vi "FFT_Austin.vi"() -> ()   [LabVIEW 2021]
uses:
  <vilib>/rvi/DataTransferAndStorage/Container/XNode/niFpgaContainer.xnode
  <vilib>/rvi/interface/RandomDataEmulation/nirviRandomDataFpgaReadWriteTemplate.vi
  <vilib>/rvi/Analysis/measure/FFT/XNode/niFpgaFFT.xnode
  <vilib>/rvi/LocalResourceManager/LocalResourceManager.xnode
  <vilib>/rvi/DataTransferAndStorage/Container/Common/niFpgaContainerGetUniqueNameForEmu.vi
  <vilib>/rvi/DataTransferAndStorage/Container/Common/niFpgaContainerSetEmuInfo.vi
  <vilib>/rvi/eio/common/nirviEmuReportErrorAndStop.vi
  <vilib>/rvi/FIFO/Fifo_Resource/niFpgaFifoEmulationRefIn.vi
  <vilib>/fxp/LVFixedPointQuantizationPolicyTypeDef.ctl
  <vilib>/rvi/Analysis/measure/FFT/simModelSupport/niFpgaFFTSimDfxp.ctl
  <vilib>/rvi/Analysis/measure/FFT/simModelSupport/niFpgaFFTSimArithmeticProperties.ctl
  <vilib>/rvi/Analysis/measure/FFT/simModelSupport/niFPGA FFT Sim Types.ctl
  <vilib>/rvi/Analysis/measure/FFT/simModelSupport/niFPGA FFT Outside SCTL Sim Properties.ctl
  <vilib>/rvi/Analysis/measure/FFT/simModelSupport/niFpgaFFTSimModelOutsideSCTLCore.vi
  <vilib>/rvi/FXPMathLib/FxpAtan2/XNode/nifxpmath_Atan2.xnode
  <vilib>/rvi/FXPMathLib/FxpAtan2/simVIs/DllFxpAtan2Temp_sub.vi
  <vilib>/rvi/FXPMathLib/FxpAtan2/subVIs/nifxpmath_Atan2_SimConfig.ctl
  <vilib>/rvi/FXPMathLib/FxpSinAndCos/subVIs/nifxpmath_SinAndCos_SimConfig.ctl
  <vilib>/rvi/FXPMathLib/FxpSinAndCos/simVIs/DllFxpSinAndCosTemp_sub.vi
  <vilib>/rvi/FXPMathLib/FxpSinAndCos/XNode/nifxpmath_SinAndCos.xnode
  <vilib>/rvi/FXPMathLib/basic elements/FxpIntAccumulator/XNode/nifxpmath_IntAccumulator.xnode
  <vilib>/rvi/FXPMathLib/basic elements/FxpIntAccumulator/simVIs/DllFxpIntAccumulator_sub.vi
  <vilib>/rvi/FXPMathLib/basic elements/FxpIntAccumulator/subVIs/nifxpmath_IntAccumulator_SimConfig.ctl
panel:
  out "Array 2":fxp<+/-,32,16>[](array[numeric])
  out "Array":fxp<+,32,16>[](array[numeric])
  out "Numeric 4":i32
  out "Numeric 3":i32
  out "Numeric":i32
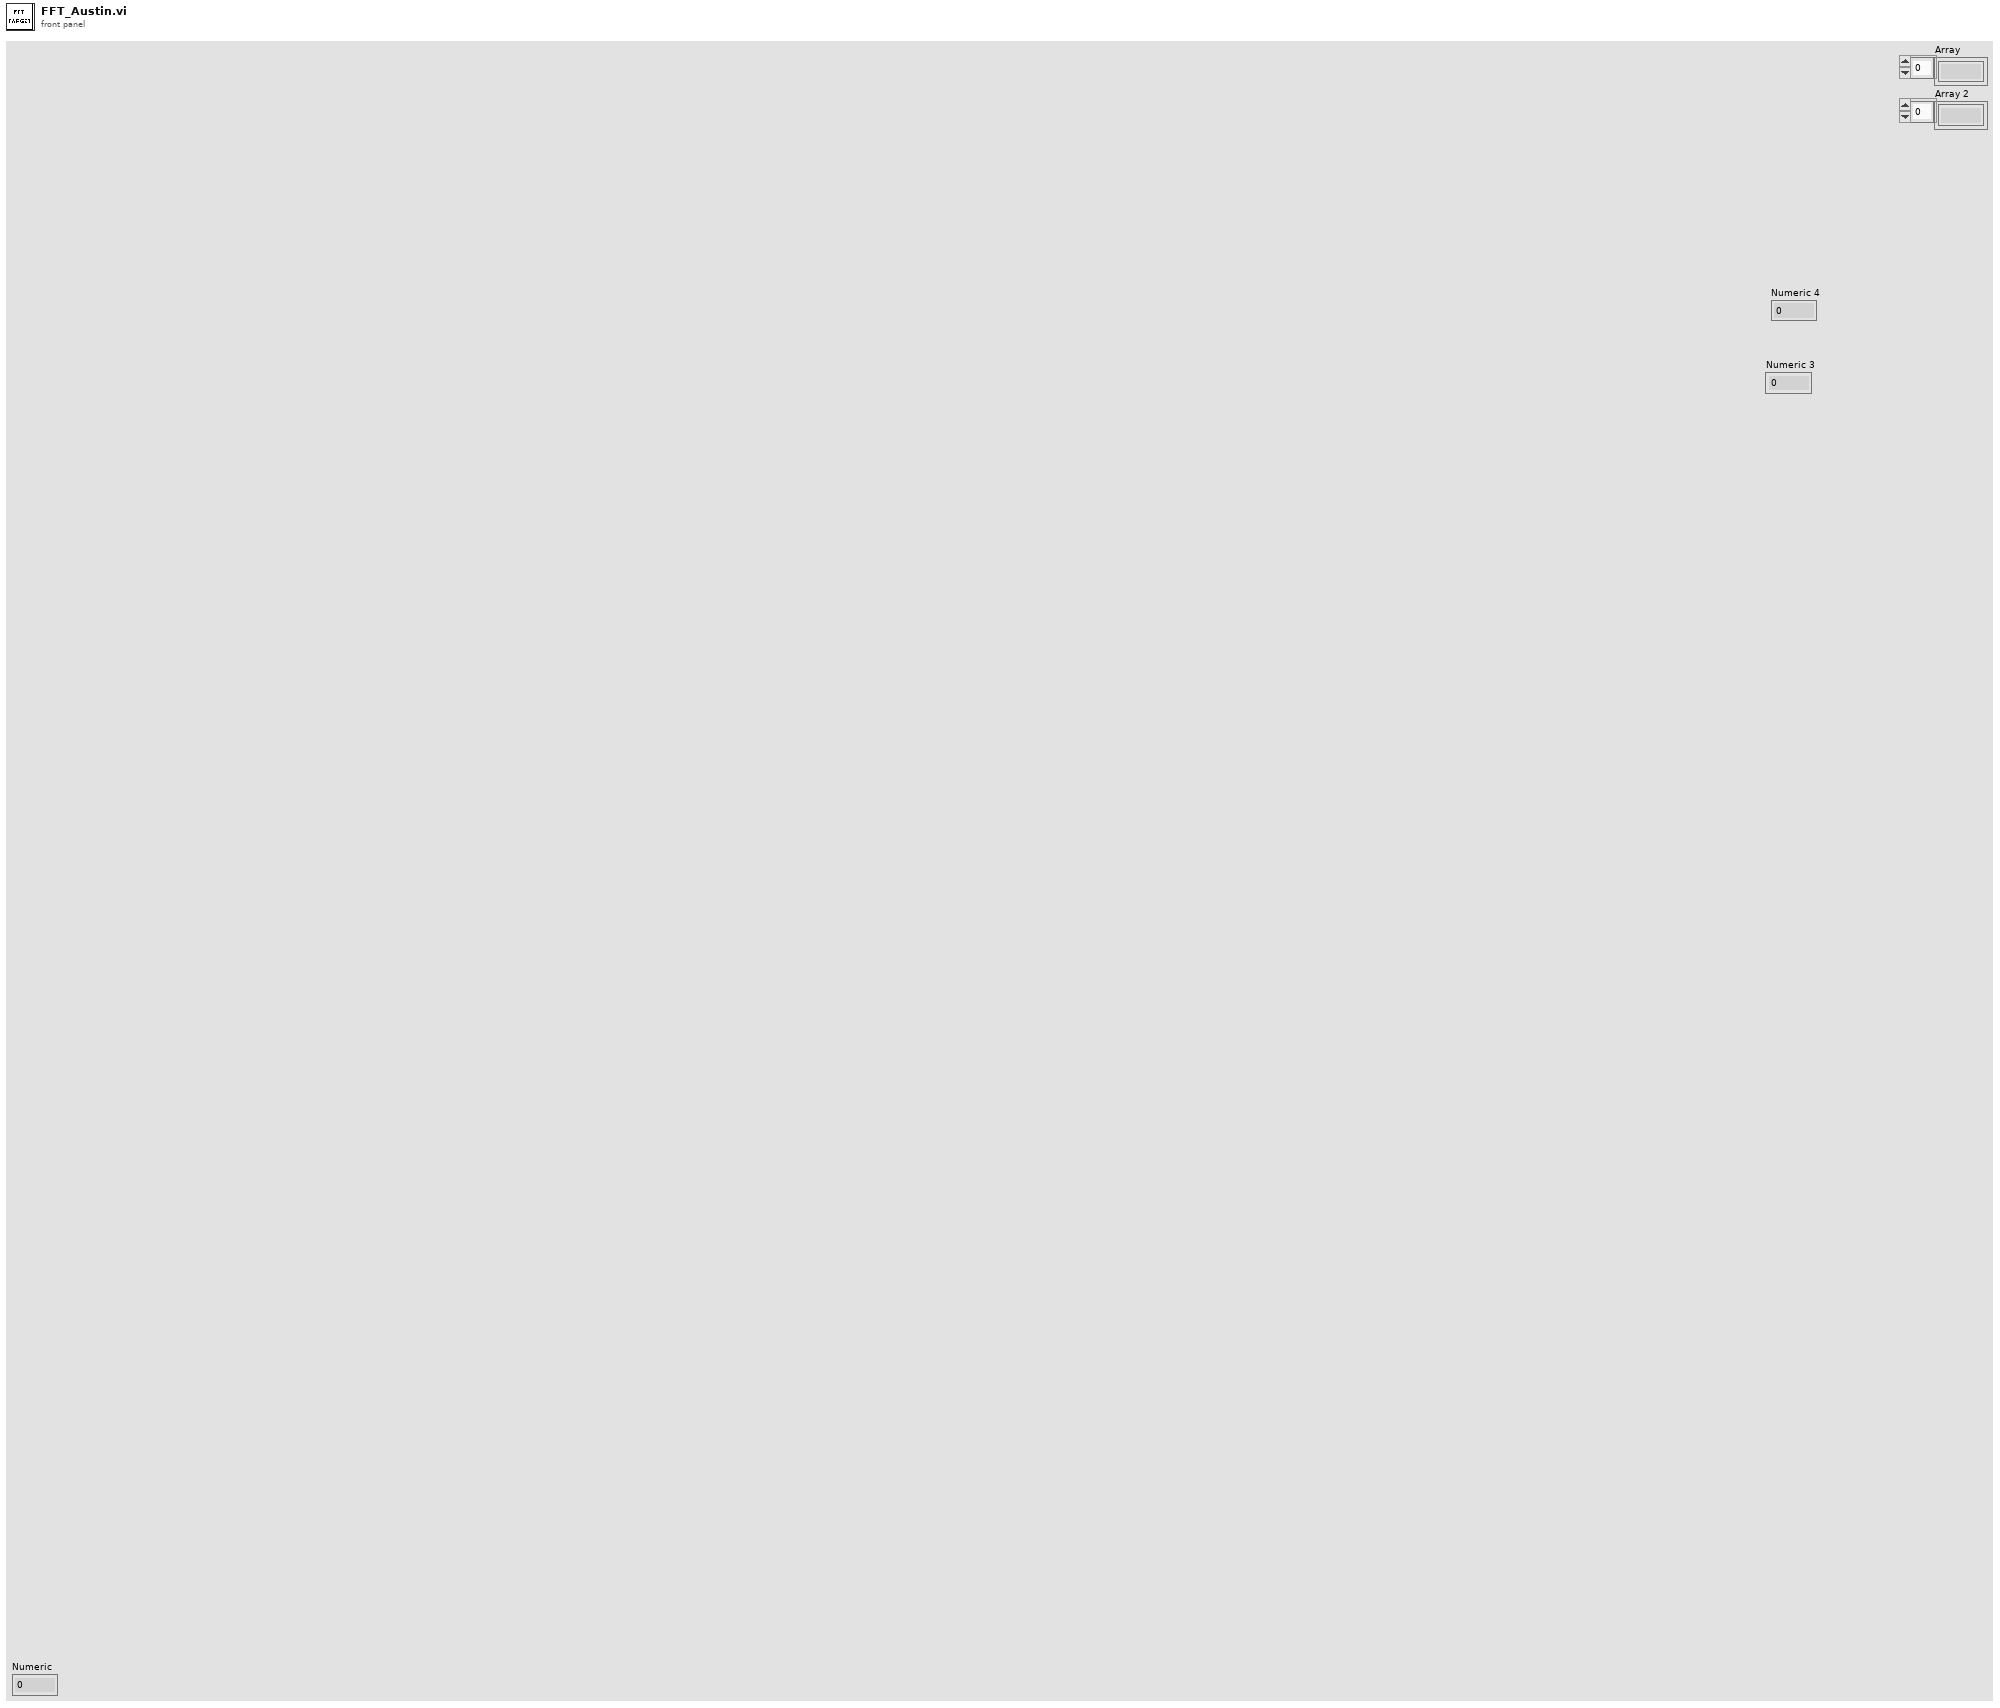
[diagram p1: front panel]
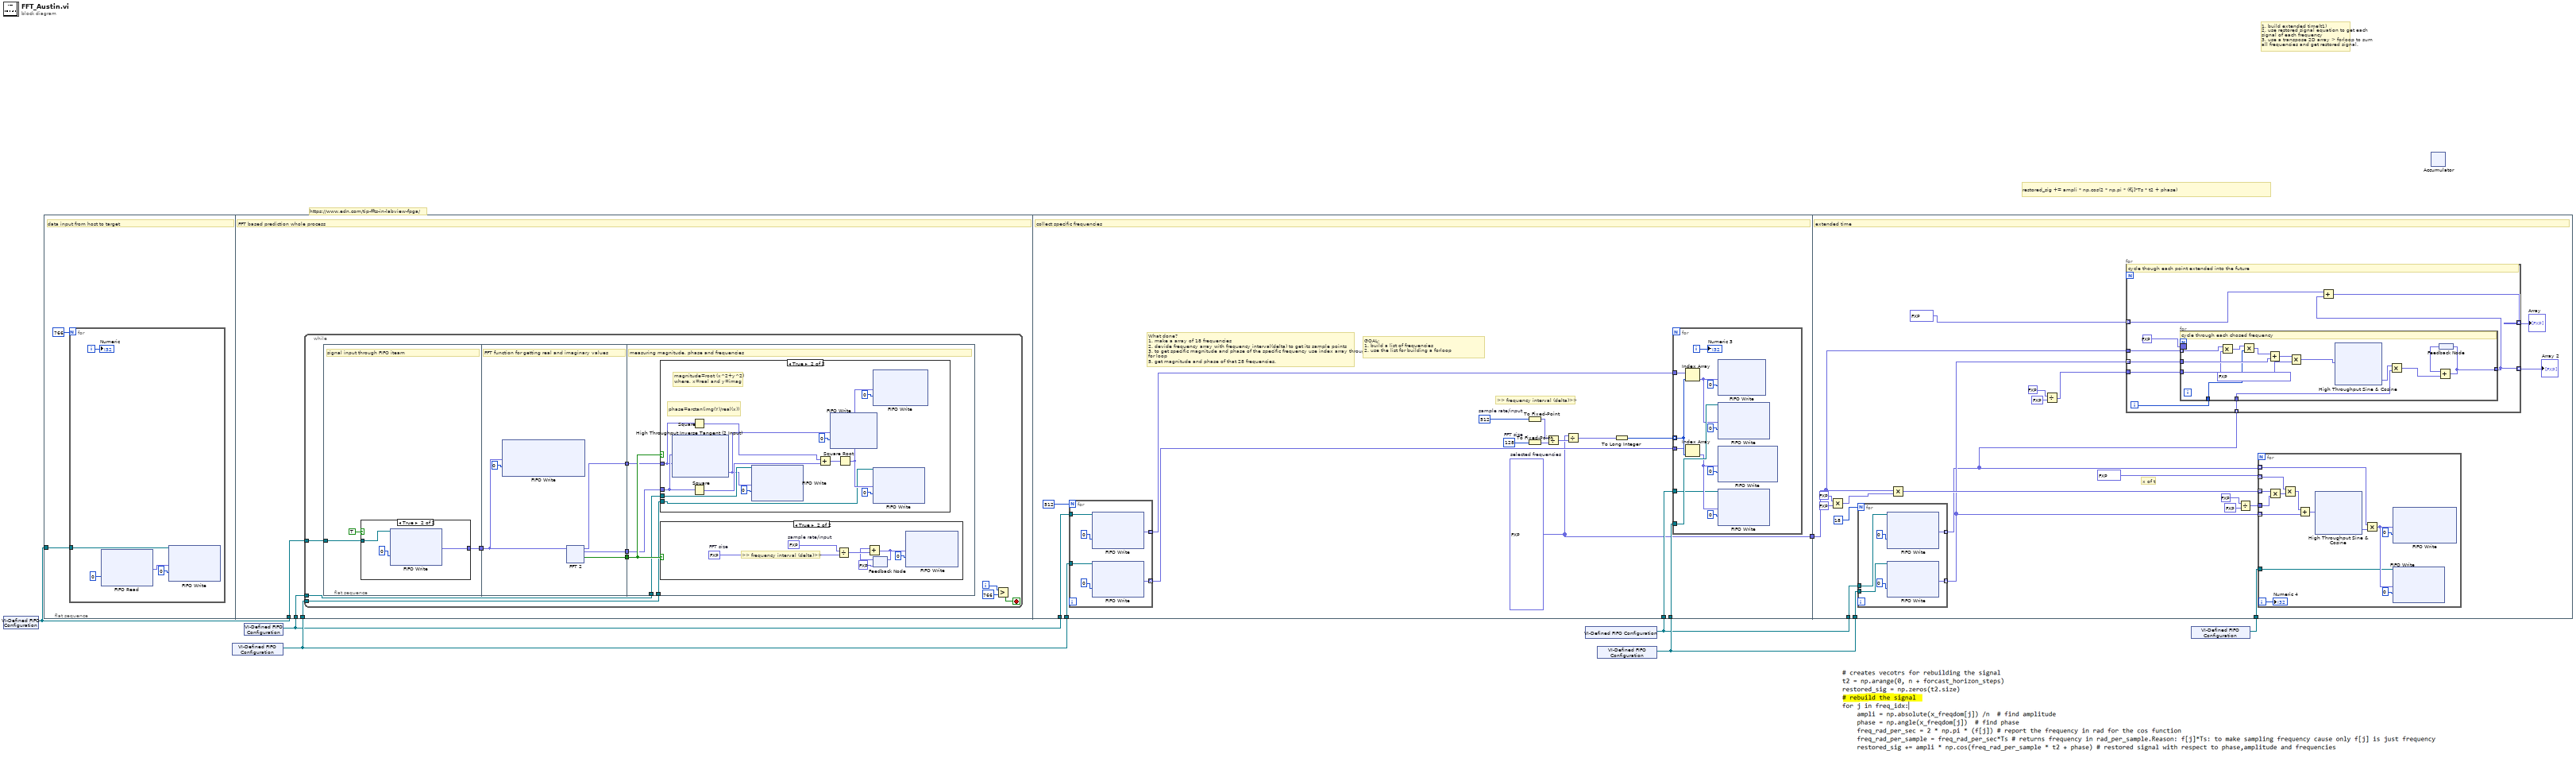
[diagram p0: block diagram]
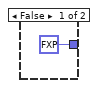
[diagram p2: hidden frame]
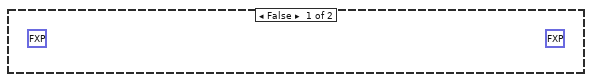
[diagram p4: hidden frame]
diagram:
  # "1. build extended time(t1)\n2. use restored signal equation to get each signal of each frequency\n3. use a transpose 2D array > forloop to sum all frequencies and get restored signal."
  # "restored_sig += ampli * np.cos(2 * np.pi * (f[j]*Ts * t2 + phase)"
  # "https://www.edn.com/tip-ffts-in-labview-fpga/"
  n1 = xnode "VI-Defined FIFO Configuration"() -> ("FIFO Out"=w7:refnum<k21>)
  n2 = flat-sequence {
    tunnel: w7 -> [w9]
    tunnel: w7 -> [w17]
    tunnel: w6 -> [w16]
    tunnel: w5 -> [w15]
    tunnel: w6 -> [w117]
    tunnel: w5 -> [w116]
    tunnel: w4 -> [w115]
    tunnel: w3 -> [w114]
    tunnel: [w113] -> w2
    tunnel: w4 -> [w166]
    tunnel: w3 -> [w165]
    tunnel: w2 -> [w151]
    tunnel: w1 -> [w159]
    frame #0 {
      # "data input from host to target"
      n3 = for {
        N: 766 -> [_]
        tunnel: w9 -> [w13]
        i -> [w10]
        n4 = xnode ("FIFO Read")("Timeout"=0) -> ("Element"=w11:fxp<+/-,24,7>)  [unwired: 1 in, 2 out]
        n5 = xnode ("FIFO Write")("Element"=w11, "Timeout"=0, "FIFO In"=w13) -> ()  [unwired: 2 out]
        "Numeric" <- w10
      }
    }
    frame #1 {
      # "FFT based prediction whole process"
      n6 = while {
        tunnel: w17 -> [w26]
        tunnel: w16 -> [w19]
        tunnel: w15 -> [w18]
        i -> [w25]
        stop <- w20 stop-if-true
        n7 = flat-sequence {
          tunnel: w26 -> [w30]
          tunnel: [w28] -> w24
          tunnel: w24 -> [w39]
          tunnel: [w38] -> w23
          tunnel: [w37] -> w22
          tunnel: [w36] -> w21
          tunnel: w23 -> [w63]
          tunnel: w22 -> [w62]
          tunnel: w21 -> [w64]
          tunnel: w19 -> [w61]
          tunnel: w18 -> [w60]
          frame #0 {
            # "signal input through FIFO iteam"
            n8 = case shown="True" TRUE {
              tunnel: w30 -> [_ w34]
              tunnel: [fxp<+/-,24,7> 0.0 ("Element") w32] -> w28
              frame False {
              }
              frame True {
                n9 = xnode ("FIFO Write")("Timeout"=0, "FIFO In"=w34) -> ("Element"=w32:fxp<+/-,24,7>)  [unwired: 2 out]
              }
            }
          }
          frame #1 {
            # "FFT function for getting real and imaginary values"
            n10 = xnode ("FIFO Write")("Element"=w39, "Timeout"=0) -> ()  [unwired: 1 in, 2 out]
            n11 = xnode ("FFT 2")("real data in"=w39) -> ("real data out"=w38:fxp<+/-,32,15>, "imaginary data out"=w37:fxp<+/-,32,15>, "output valid"=w36:bool)  [unwired: 2 in, 1 out]
          }
          frame #2 {
            # "measuring magnitude, phase and frequencies"
            n12 = case shown="True" w64 {
              tunnel: w62 -> [_ w74]
              tunnel: w63 -> [_ w73]
              tunnel: w61 -> [_ w78]
              tunnel: w60 -> [_ w75]
              frame False {
                (unwired) fxp<+/-,32,16> 0.0
                (unwired) fxp<+/-,32,16> 0.0
              }
              frame True {
                # "magnitude=root (x^2+y^2)\nwhere, x=real and y=imag"
                # "phase=arctan(img(Y)/real(x))"
                n13 = xnode "High Throughput Inverse Tangent (2 Input)"("y"=w74, "x"=w73) -> ("atan2(y,x) (pi)"=w72:fxp<+/-,16,2>)
                n14 = Square(x=w73) -> (x^2=w82:fxp<+,63,29>)
                n15 = Square(x=w74) -> (x^2=w77:fxp<+,63,29>)
                n16 = xnode ("FIFO Write")("Element"=w72, "Timeout"=0, "FIFO In"=w75) -> ()  [unwired: 2 out]
                n17 = Add(x=w82, y=w77) -> (x+y=w81:fxp<+,64,30>)
                n18 = xnode ("FIFO Write")("Element"=w72, "Timeout"=0) -> ()  [unwired: 1 in, 2 out]
                n19 = Square Root(x=w81) -> (sqrt(x)=w80:fxp<+/-,32,16>)
                n20 = xnode ("FIFO Write")("Element"=w80, "Timeout"=0) -> ()  [unwired: 1 in, 2 out]
                n21 = xnode ("FIFO Write")("Element"=w80, "Timeout"=0, "FIFO In"=w78) -> ()  [unwired: 2 out]
              }
            }
            n22 = case shown="True" w64 {
              frame False {
              }
              frame True {
                w66 = fxp<+,1,10> 512.0  # sample rate/input
                w65 = fxp<+,1,8> 128.0  # FFT size
                # ">> frequency interval (delta)>>"
                n23 = Divide(x=w66, y=w65) -> (x/y=w70:fxp<+/-,32,16>)
                n24 = feedback #1(fxp<+/-,32,16> 0.0) -> (w68:fxp<+/-,32,16>)
                n25 = Add(x=w68, y=w70) -> (x+y=w69:fxp<+/-,32,16>)
                n26 = feedback-in #1(w69) -> ()
                n27 = xnode ("FIFO Write")("Element"=w69, "Timeout"=0) -> ()  [unwired: 1 in, 2 out]
              }
            }
          }
        }
        n28 = Greater?(x=w25, y=766 ("Timeout")) -> (0:w20:bool)
      }
    }
    frame #2 {
      w122 = 512  # sample rate/input
      w123 = 128  # FFT size
      w113 = fxp<+/-,32,16>[] [128.0, 132.0, 136.0, 252.0, 256.0, 260.0, 380.0, 384.0, 388.0, -128.0, -132.0, -136.0, -252.0, -256.0, -260.0, -380.0, -384.0, -388.0]  # selected frequencies
      # "GOAL:\n1. build a list of frequencies\n2. use the list for building a forloop"
      # "What done?\n1. make a array of 18 frequencies\n2. devide frequency array with frequency interval(delta) to get its sample points\n3. to get specific magnitude and phase of the specific frequency use index array through a for loop\n5. get magnitude and phase of that 28 frequencies."
      # ">> frequency interval (delta)>>"
      # "collect specific frequencies"
      n29 = for {
        N: 512 -> [_]
        tunnel: [w143] -> w121 mode=indexing
        tunnel: [w142] -> w120 mode=indexing
        tunnel: w117 -> [w141]
        tunnel: w116 -> [w140]
        n30 = xnode ("FIFO Write")("Timeout"=0, "FIFO In"=w140) -> ("Element"=w143:fxp<+/-,16,2>)  [unwired: 2 out]
        n31 = xnode ("FIFO Write")("Timeout"=0, "FIFO In"=w141) -> ("Element"=w142:fxp<+/-,32,16>)  [unwired: 2 out]
      }
      n32 = To Fixed-Point(number=w122) -> (fixed-point=w125:fxp<+/-,32,32>)  [unwired: 1 in]
      n33 = To Fixed-Point(number=w123) -> (fixed-point=w124:fxp<+/-,32,32>)  [unwired: 1 in]
      n34 = Divide(x=w125, y=w124) -> (x/y=w126:fxp<+/-,32,16>)
      n35 = Divide(x=w113, y=w126) -> (x/y=w127:fxp<+/-,32,16>[])
      n36 = To Long Integer(number=w127) -> (32bit integer=w119:i32[])
      n37 = for {
        tunnel: w119 -> [w138] mode=indexing
        tunnel: w121 -> [w137]
        tunnel: w120 -> [w136]
        tunnel: w115 -> [w133]
        tunnel: w114 -> [w128]
        i -> [w139]
        n38 = Index Array(array=w137, index=w138) -> (element=w132:fxp<+/-,16,2>)
        n39 = Index Array(array=w136, index=w138) -> (element=w130:fxp<+/-,32,16>)
        n40 = xnode ("FIFO Write")("Element"=w132, "Timeout"=0) -> ()  [unwired: 1 in, 2 out]
        n41 = xnode ("FIFO Write")("Element"=w132, "Timeout"=0, "FIFO In"=w133) -> ()  [unwired: 2 out]
        n42 = xnode ("FIFO Write")("Element"=w130, "Timeout"=0) -> ()  [unwired: 1 in, 2 out]
        n43 = xnode ("FIFO Write")("Element"=w130, "Timeout"=0, "FIFO In"=w128) -> ()  [unwired: 2 out]
        "Numeric 3" <- w139
      }
    }
    frame #3 {
      # "x of t"
      # "extended time"
      n44 = Multiply(x=fxp<+,1,2> 2.0, y=fxp<+,2,2> 3.0) -> (x*y=w155:fxp<+,2,3>)
      n45 = for {
        N: 18 -> [_]
        tunnel: w166 -> [w269]
        tunnel: w165 -> [w268]
        tunnel: [w265] -> w147 mode=indexing
        tunnel: [w264] -> w152 mode=indexing
        n46 = xnode ("FIFO Write")("Timeout"=0, "FIFO In"=w268) -> ("Element"=w265:fxp<+/-,32,16>)  [unwired: 2 out]
        n47 = xnode ("FIFO Write")("Timeout"=0, "FIFO In"=w269) -> ("Element"=w264:fxp<+/-,16,2>)  [unwired: 2 out]
      }
      n48 = Multiply(x=w151, y=w155) -> (x*y=w158:fxp<+/-,34,19>[])
      n49 = Divide(x=fxp<+,1,1> 1.0, y=fxp<+,1,10> 512.0 ("x")) -> (x/y=w148:fxp<+,2,-8>)
      n50 = for {
        tunnel: fxp<+,32,16>[] [0.0, 0.0, 0.0, 0.0, 0.0, 0.0, 0.0, 0.0, 0.0, 0.0, 0.0, 0.0, 0.0, 0.0, 0.0, 0.0, 0.0, 0.0, 0.0, 0.0, 0.0, 0.0, 0.0, 0.0, 0.0, 0.0, 0.0, 0.0, 0.0, 0.0, 0.0, 0.0, 0.0, 0.0, 0.0, 0.0, 0.0, 0.0, 0.0, 0.0, 0.0, 0.0, 0.0, 0.0, 0.0, 0.0, 0.0, 0.0, 0.0, 0.0, 0.0, 0.0, 0.0, 0.0, 0.0, 0.0, 0.0, 0.0, 0.0, 0.0, 0.0, 0.0, 0.0, 0.0, 0.0, 0.0, 0.0, 0.0, 0.0, 0.0, 0.0, 0.0, 0.0, 0.0, 0.0, 0.0, 0.0, 0.0, 0.0, 0.0, 0.0, 0.0, 0.0, 0.0, 0.0, 0.0, 0.0, 0.0, 0.0, 0.0, 0.0, 0.0, 0.0, 0.0, 0.0, 0.0, 0.0, 0.0, 0.0, 0.0, 0.0, 0.0, 0.0, 0.0, 0.0, 0.0, 0.0, 0.0, 0.0, 0.0, 0.0, 0.0, 0.0, 0.0, 0.0, 0.0, 0.0, 0.0, 0.0, 0.0, 0.0, 0.0, 0.0, 0.0, 0.0, 0.0, 0.0, 0.0, 0.0, 0.0, 0.0, 0.0, 0.0, 0.0, 0.0, 0.0, 0.0, 0.0, 0.0, 0.0, 0.0, 0.0, 0.0, 0.0, 0.0, 0.0, 0.0, 0.0, 0.0, 0.0, 0.0, 0.0, 0.0, 0.0, 0.0, 0.0, 0.0, 0.0, 0.0, 0.0, 0.0, 0.0, 0.0, 0.0, 0.0, 0.0, 0.0, 0.0, 0.0, 0.0, 0.0, 0.0, 0.0, 0.0, 0.0, 0.0, 0.0, 0.0, 0.0, 0.0, 0.0, 0.0, 0.0, 0.0, 0.0, 0.0, 0.0, 0.0, 0.0, 0.0, 0.0, 0.0, 0.0, 0.0, 0.0, 0.0, 0.0, 0.0, 0.0, 0.0, 0.0, 0.0, 0.0, 0.0, 0.0, 0.0, 0.0, 0.0, 0.0, 0.0, 0.0, 0.0, 0.0, 0.0, 0.0, 0.0, 0.0, 0.0, 0.0, 0.0, 0.0, 0.0, 0.0, 0.0, 0.0, 0.0, 0.0, 0.0, 0.0, 0.0, 0.0, 0.0, 0.0, 0.0, 0.0, 0.0, 0.0, 0.0, 0.0, 0.0, 0.0, 0.0, 0.0, 0.0, 0.0, 0.0, 0.0, 0.0, 0.0, 0.0, 0.0, 0.0, 0.0, 0.0, 0.0, 0.0, 0.0, 0.0, 0.0, 0.0, 0.0, 0.0, 0.0, 0.0, 0.0, 0.0, 0.0, 0.0, 0.0, 0.0, 0.0, 0.0, 0.0, 0.0, 0.0, 0.0, 0.0, 0.0, 0.0, 0.0, 0.0, 0.0, 0.0, 0.0, 0.0, 0.0, 0.0, 0.0, 0.0, 0.0, 0.0, 0.0, 0.0, 0.0, 0.0, 0.0, 0.0, 0.0, 0.0, 0.0, 0.0, 0.0, 0.0, 0.0, 0.0, 0.0, 0.0, 0.0, 0.0, 0.0, 0.0, 0.0, 0.0, 0.0, 0.0, 0.0, 0.0, 0.0, 0.0, 0.0, 0.0, 0.0, 0.0, 0.0, 0.0, 0.0, 0.0, 0.0, 0.0, 0.0, 0.0, 0.0, 0.0, 0.0, 0.0, 0.0, 0.0, 0.0, 0.0, 0.0, 0.0, 0.0, 0.0, 0.0, 0.0, 0.0, 0.0, 0.0, 0.0, 0.0, 0.0, 0.0, 0.0, 0.0, 0.0, 0.0, 0.0, 0.0, 0.0, 0.0, 0.0, 0.0, 0.0, 0.0, 0.0, 0.0, 0.0, 0.0, 0.0, 0.0, 0.0, 0.0, 0.0, 0.0, 0.0, 0.0, 0.0, 0.0, 0.0, 0.0, 0.0, 0.0, 0.0, 0.0, 0.0, 0.0, 0.0, 0.0, 0.0, 0.0, 0.0, 0.0, 0.0, 0.0, 0.0, 0.0, 0.0, 0.0, 0.0, 0.0, 0.0, 0.0, 0.0, 0.0, 0.0, 0.0, 0.0, 0.0, 0.0, 0.0, 0.0, 0.0, 0.0, 0.0, 0.0, 0.0, 0.0, 0.0, 0.0, 0.0, 0.0, 0.0, 0.0, 0.0, 0.0, 0.0, 0.0, 0.0, 0.0, 0.0, 0.0, 0.0, 0.0, 0.0, 0.0, 0.0, 0.0, 0.0, 0.0, 0.0, 0.0, 0.0, 0.0, 0.0, 0.0, 0.0, 0.0, 0.0, 0.0, 0.0, 0.0, 0.0, 0.0, 0.0, 0.0, 0.0, 0.0, 0.0, 0.0, 0.0, 0.0, 0.0, 0.0, 0.0, 0.0, 0.0, 0.0, 0.0, 0.0, 0.0, 0.0, 0.0, 0.0, 0.0, 0.0, 0.0, 0.0, 0.0, 0.0, 0.0, 0.0, 0.0, 0.0, 0.0, 0.0, 0.0, 0.0, 0.0, 0.0, 0.0, 0.0, 0.0, 0.0, 0.0, 0.0, 0.0, 0.0, 0.0, 0.0, 0.0, 0.0, 0.0, 0.0, 0.0, 0.0, 0.0, 0.0, 0.0, 0.0, 0.0, 0.0, 0.0] -> [w175] mode=indexing
        tunnel: [w174] -> w153 mode=indexing
        tunnel: w152 -> [w173] mode=indexing
        tunnel: w151 -> [w172]
        tunnel: w148 -> [w171]
        tunnel: w147 -> [w169] mode=indexing
        tunnel: [w167] -> w146 mode=indexing
        i -> [w170]
        # "cycle though each point extended into the future"
        n51 = for {
          tunnel: w173 -> [w189]
          tunnel: w172 -> [w188] mode=indexing
          tunnel: w171 -> [w187]
          tunnel: w170 -> [w185]
          tunnel: w169 -> [w179]
          border: fxp<+,1,1> 0.0 -> [_]
          tunnel: [w176] -> w167
          # "cycle through each chosed frequency"
          n52 = Multiply(x=w188, y=w187) -> (x*y=w186:fxp<+/-,33,7>)
          n53 = Multiply(x=w186, y=w185) -> (x*y=w184:fxp<+/-,64,39>)
          n54 = Add(x=w184, y=w189) -> (x+y=w183:fxp<+/-,64,40>)
          n55 = Multiply(x=w183, y=fxp<+/-,64,40> 6.283185303211212) -> (x*y=w181:fxp<+/-,64,80>)
          n56 = xnode "High Throughput Sine & Cosine"("x (pi)"=w181) -> ("cos(x)"=w180:fxp<+/-,16,2>)  [unwired: 1 out]
          n57 = Multiply(x=w180, y=w179) -> (x*y=w177:fxp<+/-,48,18>)
          n58 = feedback #2() -> (w178:fxp<+/-,32,16>)
          n59 = Add(x=w178, y=w177) -> (x+y=w176:fxp<+/-,32,16>)
          n60 = feedback-in #2(w176) -> ()
        }
        n61 = Add(x=w175, y=w167) -> (x+y=w174:fxp<+/-,34,18>)
      }
      "Array" <- w153
      "Array 2" <- w146
      n62 = Divide(x=fxp<+,1,1> 1.0, y=fxp<+,1,10> 512.0 ("x")) -> (x/y=w157:fxp<+,2,-8>)
      n63 = for {
        tunnel: w159 -> [w228]
        tunnel: w158 -> [w226] mode=indexing
        tunnel: w157 -> [w225]
        tunnel: w152 -> [w223] mode=indexing
        tunnel: w147 -> [w222] mode=indexing
        tunnel: fxp<+,32,16>[] [0.0, 0.0, 0.0, 0.0, 0.0, 0.0, 0.0, 0.0, 0.0, 0.0, 0.0, 0.0, 0.0, 0.0, 0.0, 0.0, 0.0, 0.0, 0.0, 0.0, 0.0, 0.0, 0.0, 0.0, 0.0, 0.0, 0.0, 0.0, 0.0, 0.0, 0.0, 0.0, 0.0, 0.0, 0.0, 0.0, 0.0, 0.0, 0.0, 0.0, 0.0, 0.0, 0.0, 0.0, 0.0, 0.0, 0.0, 0.0, 0.0, 0.0, 0.0, 0.0, 0.0, 0.0, 0.0, 0.0, 0.0, 0.0, 0.0, 0.0, 0.0, 0.0, 0.0, 0.0, 0.0, 0.0, 0.0, 0.0, 0.0, 0.0, 0.0, 0.0, 0.0, 0.0, 0.0, 0.0, 0.0, 0.0, 0.0, 0.0, 0.0, 0.0, 0.0, 0.0, 0.0, 0.0, 0.0, 0.0, 0.0, 0.0, 0.0, 0.0, 0.0, 0.0, 0.0, 0.0, 0.0, 0.0, 0.0, 0.0, 0.0, 0.0, 0.0, 0.0, 0.0, 0.0, 0.0, 0.0, 0.0, 0.0, 0.0, 0.0, 0.0, 0.0, 0.0, 0.0, 0.0, 0.0, 0.0, 0.0, 0.0, 0.0, 0.0, 0.0, 0.0, 0.0, 0.0, 0.0, 0.0, 0.0, 0.0, 0.0, 0.0, 0.0, 0.0, 0.0, 0.0, 0.0, 0.0, 0.0, 0.0, 0.0, 0.0, 0.0, 0.0, 0.0, 0.0, 0.0, 0.0, 0.0, 0.0, 0.0, 0.0, 0.0, 0.0, 0.0, 0.0, 0.0, 0.0, 0.0, 0.0, 0.0, 0.0, 0.0, 0.0, 0.0, 0.0, 0.0, 0.0, 0.0, 0.0, 0.0, 0.0, 0.0, 0.0, 0.0, 0.0, 0.0, 0.0, 0.0, 0.0, 0.0, 0.0, 0.0, 0.0, 0.0, 0.0, 0.0, 0.0, 0.0, 0.0, 0.0, 0.0, 0.0, 0.0, 0.0, 0.0, 0.0, 0.0, 0.0, 0.0, 0.0, 0.0, 0.0, 0.0, 0.0, 0.0, 0.0, 0.0, 0.0, 0.0, 0.0, 0.0, 0.0, 0.0, 0.0, 0.0, 0.0, 0.0, 0.0, 0.0, 0.0, 0.0, 0.0, 0.0, 0.0, 0.0, 0.0, 0.0, 0.0, 0.0, 0.0, 0.0, 0.0, 0.0, 0.0, 0.0, 0.0, 0.0, 0.0, 0.0, 0.0, 0.0, 0.0, 0.0, 0.0, 0.0, 0.0, 0.0, 0.0, 0.0, 0.0, 0.0, 0.0, 0.0, 0.0, 0.0, 0.0, 0.0, 0.0, 0.0, 0.0, 0.0, 0.0, 0.0, 0.0, 0.0, 0.0, 0.0, 0.0, 0.0, 0.0, 0.0, 0.0, 0.0, 0.0, 0.0, 0.0, 0.0, 0.0, 0.0, 0.0, 0.0, 0.0, 0.0, 0.0, 0.0, 0.0, 0.0, 0.0, 0.0, 0.0, 0.0, 0.0, 0.0, 0.0, 0.0, 0.0, 0.0, 0.0, 0.0, 0.0, 0.0, 0.0, 0.0, 0.0, 0.0, 0.0, 0.0, 0.0, 0.0, 0.0, 0.0, 0.0, 0.0, 0.0, 0.0, 0.0, 0.0, 0.0, 0.0, 0.0, 0.0, 0.0, 0.0, 0.0, 0.0, 0.0, 0.0, 0.0, 0.0, 0.0, 0.0, 0.0, 0.0, 0.0, 0.0, 0.0, 0.0, 0.0, 0.0, 0.0, 0.0, 0.0, 0.0, 0.0, 0.0, 0.0, 0.0, 0.0, 0.0, 0.0, 0.0, 0.0, 0.0, 0.0, 0.0, 0.0, 0.0, 0.0, 0.0, 0.0, 0.0, 0.0, 0.0, 0.0, 0.0, 0.0, 0.0, 0.0, 0.0, 0.0, 0.0, 0.0, 0.0, 0.0, 0.0, 0.0, 0.0, 0.0, 0.0, 0.0, 0.0, 0.0, 0.0, 0.0, 0.0, 0.0, 0.0, 0.0, 0.0, 0.0, 0.0, 0.0, 0.0, 0.0, 0.0, 0.0, 0.0, 0.0, 0.0, 0.0, 0.0, 0.0, 0.0, 0.0, 0.0, 0.0, 0.0, 0.0, 0.0, 0.0, 0.0, 0.0, 0.0, 0.0, 0.0, 0.0, 0.0, 0.0, 0.0, 0.0, 0.0, 0.0, 0.0, 0.0, 0.0, 0.0, 0.0, 0.0, 0.0, 0.0, 0.0, 0.0, 0.0, 0.0, 0.0, 0.0, 0.0, 0.0, 0.0, 0.0, 0.0, 0.0, 0.0, 0.0, 0.0, 0.0, 0.0, 0.0, 0.0, 0.0, 0.0, 0.0, 0.0, 0.0, 0.0, 0.0, 0.0, 0.0, 0.0, 0.0, 0.0, 0.0, 0.0, 0.0, 0.0, 0.0, 0.0, 0.0, 0.0, 0.0, 0.0, 0.0, 0.0, 0.0, 0.0, 0.0, 0.0, 0.0, 0.0, 0.0, 0.0, 0.0, 0.0, 0.0, 0.0, 0.0, 0.0, 0.0, 0.0, 0.0, 0.0, 0.0, 0.0, 0.0, 0.0, 0.0, 0.0, 0.0, 0.0, 0.0, 0.0, 0.0, 0.0, 0.0, 0.0, 0.0, 0.0, 0.0, 0.0, 0.0] -> [w221] mode=indexing
        i -> [w220]
        n64 = Multiply(x=w226, y=w225) -> (x*y=w224:fxp<+/-,32,16>)
        n65 = Multiply(x=w221, y=w224) -> (x*y=w233:fxp<+/-,32,16>)
        n66 = Add(x=w233, y=w223) -> (x+y=w227:fxp<+/-,32,16>)
        n67 = xnode "High Throughput Sine & Cosine"("x (pi)"=w227) -> ("cos(x)"=w232:fxp<+/-,32,2>)  [unwired: 1 out]
        n68 = Multiply(x=w222, y=w232) -> (x*y=w230:fxp<+/-,64,18>)
        n69 = xnode ("FIFO Write")("Element"=w230, "Timeout"=0) -> ()  [unwired: 1 in, 2 out]
        n70 = xnode ("FIFO Write")("Element"=w230, "Timeout"=0, "FIFO In"=w228) -> ()  [unwired: 2 out]
        "Numeric 4" <- w220
      }
    }
  }
  n71 = xnode "VI-Defined FIFO Configuration"() -> ("FIFO Out"=w6:refnum<k21>)
  n72 = xnode "VI-Defined FIFO Configuration"() -> ("FIFO Out"=w5:refnum<k21>)
  n73 = xnode "VI-Defined FIFO Configuration"() -> ("FIFO Out"=w3:refnum<k21>)
  n74 = xnode "VI-Defined FIFO Configuration"() -> ("FIFO Out"=w4:refnum<k21>)
  n75 = xnode "VI-Defined FIFO Configuration"() -> ("FIFO Out"=w1:refnum<k21>)
  n76 = xnode "Accumulator"() -> ()  [unwired: 5 in, 2 out]
